vi "Create CallerWatchdog Queue.vi"(8 "error in (no error)":errorcluster, 11 "SMO in":refnum<class "SMO.lvclass">) -> (0 "error out":errorcluster, 3 "SMO out":refnum<class "SMO.lvclass">)   [LabVIEW 2013, in "SMO.lvclass"]
uses:
  SMO.lvclass
  SMO.lvclass/SMO.ctl
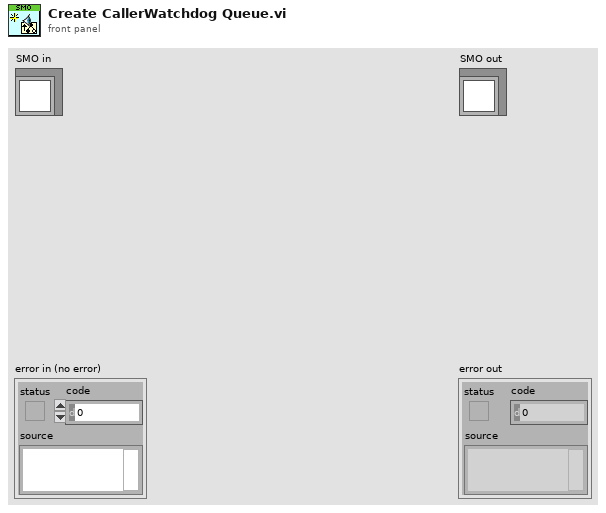
[diagram p1: front panel]
types:
  T1 = typedef "SMO.lvclass/PrivateData--Ref.ctl" = refnum<data-value>
  T2 = typedef "SMO.lvclass/PrivateData--Cluster.ctl" = cluster{"Parent Call":T3, "Registered Processes":T4[], "Sync Notifier":refnum<notifier>, "Process Error Notifier":refnum<notifier>, "Protected Events":T5, "Public Events":T6, "SMO State":T7, "[Attributes]":variant, "Launcher Close":refnum<notifier>, "Caller Watchdog":refnum<queue>, "Accessibility":T8, "NbStaticDependencies":u32}
  T3 = typedef "SMO.lvclass/Parent Call--Enum.ctl" = enum16{"Allows parent to run", "Does not request parent to run"}
  T4 = typedef "SMO.lvclass/RegisteredProcessData--Cluster.ctl" = cluster{"Name":string, "Static VI Ref":refnum<vi>, "Running":bool, "NotifierRef":u32}
  T5 = typedef "SMO.lvclass/Protected Events.ctl" = cluster{"StopProcesses":refnum<user-event>, "AbortProcesses":refnum<user-event>, "Config Changed":refnum<user-event>, "Dependency":refnum<user-event>}
  T6 = typedef "SMO.lvclass/Public Events.ctl" = cluster{"Error":refnum<user-event>, "State":refnum<user-event>, "Reserve State":refnum<user-event>}
  T7 = typedef "SMO.lvclass/SMOState --Enum.ctl" = enum16{"unknown", "Created", "Started", "Stopped"}
  T8 = typedef "SMO.lvclass/Accessibility--Cluster.ctl" = cluster{"Lock Key":string, "Reserve State":T9}
  T9 = typedef "SMO.lvclass/Reserve State--Enum.ctl" = enum16{"Unreserved", "Reserved", "Self-locked"}
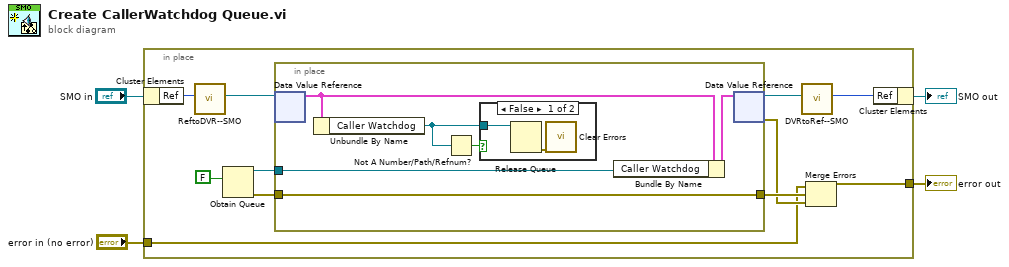
[diagram p0: block diagram]
diagram:
  n1 = in-place {
    in-place-border: "error in (no error)" -> [w6]
    in-place-border: [w5] -> w1
    n2 = in-place-cluster #1("SMO in") -> ("Ref"=w14:u32)
    n3 = call "ReftoDVR--SMO.vi"("Ref"=w14) -> ("Ref"=w12:T1)  [unwired: 10 in]
    n4 = Obtain Queue(element data type=FALSE) -> (queue out=w11:refnum<queue>, error out=w9:errorcluster)  [unwired: 4 in, 1 out]
    n5 = in-place {
      in-place-border: w11 -> [w21]
      in-place-border: w9 -> [w19]
      in-place-border: [w19] -> w8
      n6 = in-place-dvr #2(w12) -> (w18:T2)  [unwired: 1 out]
      n7 = Unbundle By Name(w18) -> ("Caller Watchdog"=w17:refnum<queue>)
      n8 = Not A Number/Path/Refnum?(number/path/refnum=w17) -> (NaN/Path/Refnum?=w16:bool)
      n9 = case shown="False" w16 {
        tunnel: w17 -> [w22 _]
        frame False {
          n10 = Release Queue(queue=w22) -> (error out=w23:errorcluster)  [unwired: 2 in, 2 out]
          n11 = call <vilib>:"Clear Errors.vi"("error in (no error)"=w23) -> ()  [unwired: 6 in, 1 out]
        }
        frame True {
        }
      }
      n12 = Bundle By Name(cluster=w18, "Caller Watchdog"=w21) -> (w20:T2)
      n13 = in-place-dvr #2(w20) -> (w10:T1, w7:errorcluster)
    }
    n14 = call "DVRtoRef--SMO.vi"("Ref"=w10) -> ("Ref"=w13:u32)  [unwired: 10 in]
    n15 = Merge Errors(w6, w8, w7) -> (w5:errorcluster)
    n16 = in-place-cluster #1("Ref"=w13) -> (→"SMO out":refnum<class "SMO.lvclass">)
  }
  "error out" <- w1
